vi "физ6.vi"() -> ()   [LabVIEW 2021]
panel:
  out "Количество теплоты":dbl
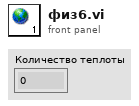
[diagram p1: front panel]
diagram:
